vi "Close.vi"(8 "error in":errorcluster, 11 "Chiller Cluster - 2 Channel.lvclass":refnum<class "Chiller Cluster - 2 Channel.lvclass">) -> (0 "error out":errorcluster)   [LabVIEW 2023, in "Chiller Cluster - 2 Channel.lvclass"]
uses:
  Chiller Cluster - 2 Channel.lvclass
  Chiller Cluster - 2 Channel.lvclass/Chiller Cluster - 2 Channel.ctl
  <vilib>/ADAS Replay HIL/AdasHilServices/AdasHilServices Fill In Error Info Ex.vi
  <vilib>/ADAS Replay HIL/AdasHilServices/AdasHilChannelServices.lvlib
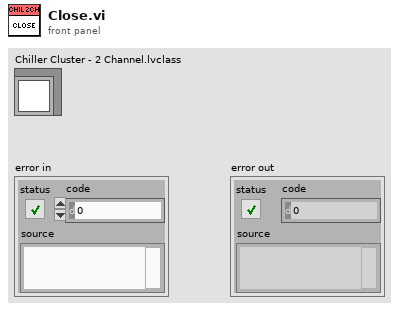
[diagram p1: front panel]
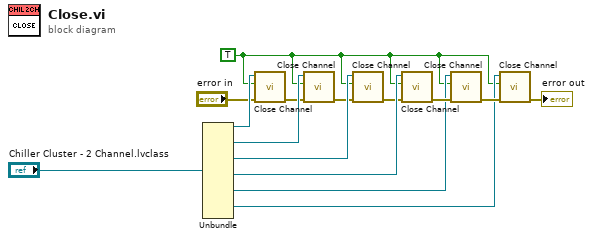
[diagram p0: block diagram]
diagram:
  w1 = TRUE ("Force Destroy? (F)")
  n1 = Unbundle("Chiller Cluster - 2 Channel.lvclass") -> (w15:refnum<k21>, w14:refnum<k21>, w11:refnum<k21>, w10:refnum<k21>, w3:refnum<k21>, w2:refnum<k21>)  [unwired: 6 out]
  n2 = call <vilib>:"Close Channel.vi"("error in"="error in", "Force Destroy? (F)"=w1, "ADAS HIL Channel"=w15) -> ("error out"=w12:errorcluster)  [unwired: 8 in]
  n3 = call <vilib>:"Close Channel.vi"("error in"=w12, "Force Destroy? (F)"=w1, "ADAS HIL Channel"=w14) -> ("error out"=w9:errorcluster)  [unwired: 8 in]
  n4 = call <vilib>:"Close Channel.vi"("error in"=w9, "Force Destroy? (F)"=w1, "ADAS HIL Channel"=w11) -> ("error out"=w8:errorcluster)  [unwired: 8 in]
  n5 = call <vilib>:"Close Channel.vi"("error in"=w8, "Force Destroy? (F)"=w1, "ADAS HIL Channel"=w10) -> ("error out"=w6:errorcluster)  [unwired: 8 in]
  n6 = call <vilib>:"Close Channel.vi"("error in"=w6, "Force Destroy? (F)"=w1, "ADAS HIL Channel"=w3) -> ("error out"=w5:errorcluster)  [unwired: 8 in]
  n7 = call <vilib>:"Close Channel.vi"("error in"=w5, "Force Destroy? (F)"=w1, "ADAS HIL Channel"=w2) -> ("error out"=→"error out":errorcluster)  [unwired: 8 in]
